vi "Bulk Update Description.vi"() -> ()   [LabVIEW 2023]
panel:
  out "VI Name":string
  out "concatenated string":string
  out "error out":errorcluster
  in  "Root Directory":path
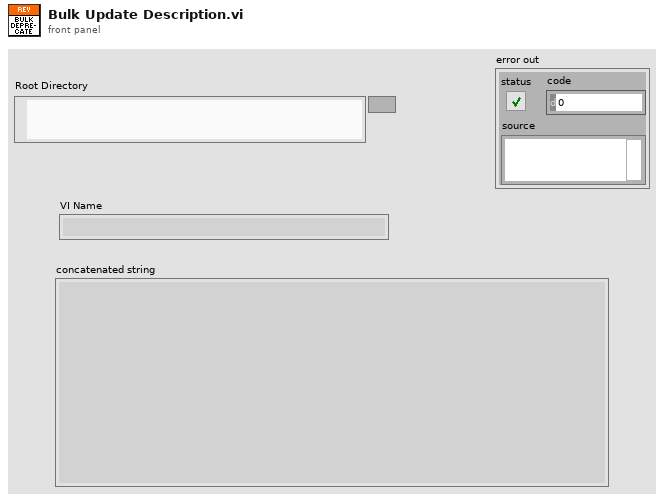
[diagram p1: front panel]
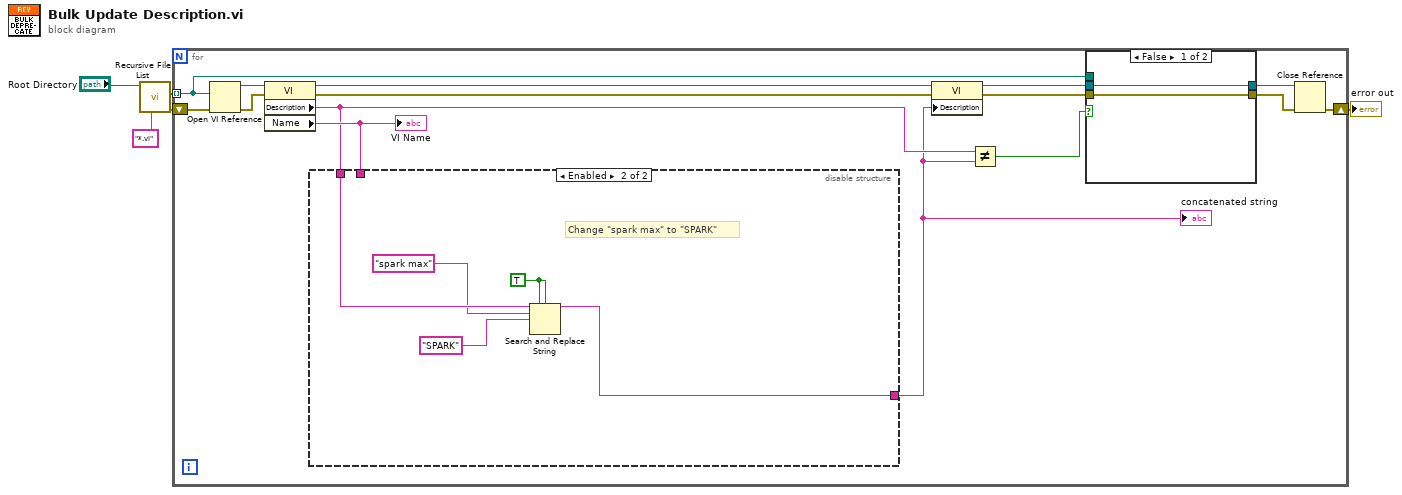
[diagram p0: block diagram]
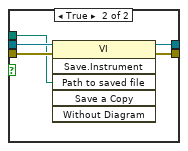
[diagram p2: hidden frame]
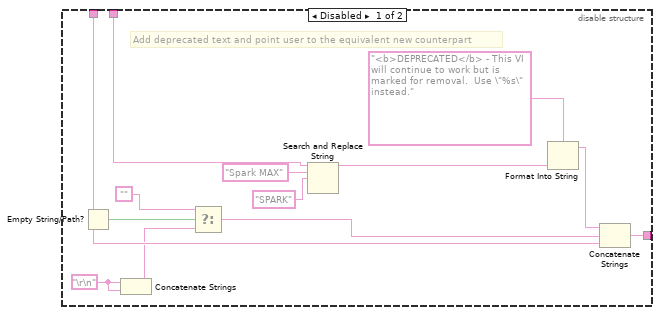
[diagram p3: hidden frame]
diagram:
  n1 = call <vilib>:"Recursive File List.vi"("pattern"="*.vi", "Folder Path"="Root Directory") -> ("error out"=w3:errorcluster, "All Files in Dir"=w4:path[])  [unwired: 5 in, 3 out]
  n2 = for {
    tunnel: w4 -> [w9] mode=indexing
    shift-right: [w15] -> w1
    shift-left: w3 -> [w20]
    n3 = Open VI Reference(vi path=w9, error in (no error)=w20) -> (vi reference=w19:refnum<vi>, error out=w18:errorcluster)  [unwired: 4 in]
    n4 = property class="VI"(reference=w19, error in=w18) -> (reference out=w17:refnum<vi>, error out=w16:errorcluster, "Description"=w8:string, "Name"=w14:string)
    "VI Name" <- w14
    n5 = disable-structure shown="Enabled" {
      disable-tunnel: w8 -> [w37 w45]
      disable-tunnel: w14 -> [w32 _]
      disable-tunnel: [w30 w42] -> w7
      frame Disabled {
        w36 = "\r\n"
        # "Add deprecated text and point user to the equivalent new counterpart"
        n6 = Empty String/Path?(string/path=w37) -> (empty?=w40:bool)
        n7 = Concatenate Strings(w36, w36) -> (w35:string)
        n8 = Select(t="", s=w40, f=w35) -> (s? t:f=w38:string)
        n9 = Search and Replace String(input string=w32, search string="Spark MAX", replace string="SPARK" ("replace string (\"\")")) -> (result string=w31:string)  [unwired: 5 in, 3 out]
        n10 = Format Into String(format string="<b>DEPRECATED</b> - This VI will continue to work but is marked for removal.  Use \"%s\" instead." ("pattern"), w31) -> (resulting string=w34:string)  [unwired: 2 in, 1 out]
        n11 = Concatenate Strings(w34, w38, w37) -> (w30:string)
      }
      frame Enabled {
        w41 = TRUE ("ignore case? (F)")
        # "Change \"spark max\" to \"SPARK\""
        n12 = Search and Replace String(replace all?=w41, case sensitive?=w41, input string=w45, search string="spark max", replace string="SPARK" ("replace string (\"\")")) -> (result string=w42:string)  [unwired: 3 in, 3 out]
      }
    }
    "concatenated string" <- w7
    n13 = property class="VI"(reference=w17, error in=w16, "Description"=w7) -> (reference out=w13:refnum<vi>, error out=w11:errorcluster)
    n14 = Not Equal?(x=w8, y=w7) -> (x != y?=w6:bool)
    n15 = case shown="False" w6 {
      tunnel: w13 -> [w21 w27]
      tunnel: [w21 w26] -> w12
      tunnel: w11 -> [w22 w25]
      tunnel: [w22 w24] -> w10
      tunnel: w9 -> [_ w23]
      frame False {
      }
      frame True {
        n16 = invoke class="VI" method="Save.Instrument"(reference=w27, error in=w25, "Path to saved file"=w23) -> (reference out=w26:refnum<vi>, error out=w24:errorcluster)  [unwired: 3 in, 4 out]
      }
    }
    n17 = Close Reference(reference=w12, error in (no error)=w10) -> (error out=w15:errorcluster)
  }
  "error out" <- w1
